vi "ALTS-2015 Show Remaining Time .vi"(8 "error in (no error)":errorcluster, 11 "Time Delay to Restart (Mins)":dbl=2.0 format="%#_13g") -> (0 "error out":errorcluster)   [LabVIEW 2013]
panel:
  in  "Jump Button":bool
  out "Time to be elapsed (in seconds)":u32
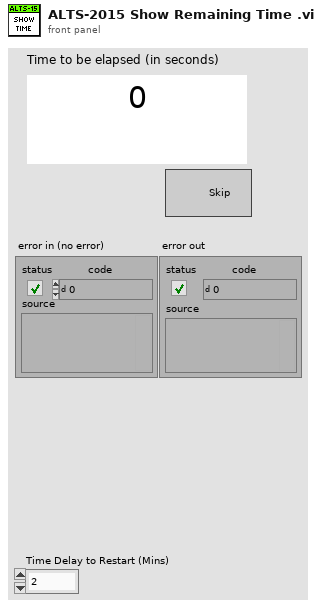
[diagram p1: front panel]
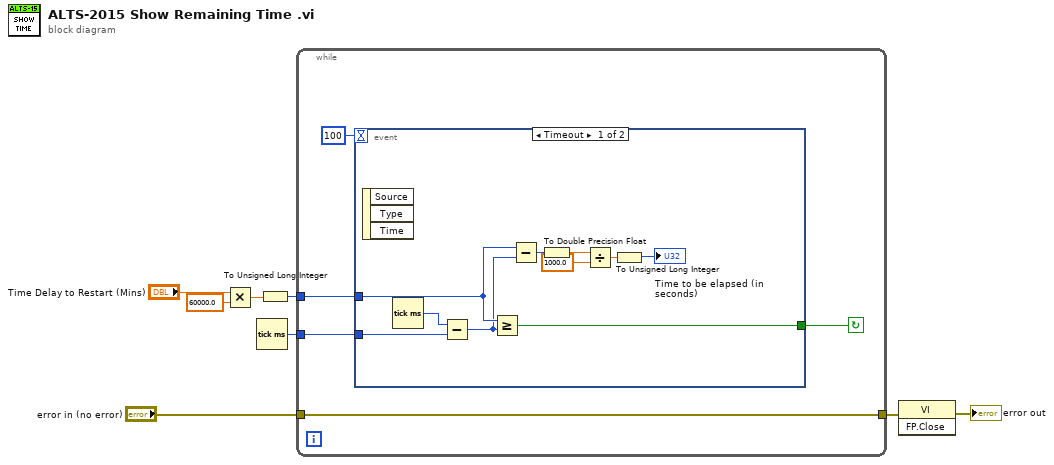
[diagram p0: block diagram]
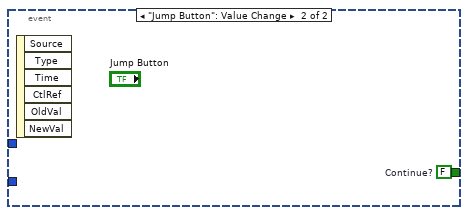
[diagram p2: hidden frame]
diagram:
  n1 = Multiply(x="Time Delay to Restart (Mins)", y=60000.0) -> (x*y=w5:dbl)
  n2 = Tick Count (ms)() -> (millisecond timer value=w8:u32)
  n3 = To Unsigned Long Integer(number=w5) -> (unsigned 32bit integer=w4:u32)
  n4 = while {
    tunnel: w8 -> [w12]
    tunnel: w4 -> [w11]
    tunnel: "error in (no error)" -> [w9]
    tunnel: [w9] -> w3
    stop <- w10 continue-if-true
    n5 = event shown="[0] Timeout" {
      selector: _ -> [_ _]
      dyn-events: _ -> [_ _]
      timeout: 100 -> [_ _]
      tunnel: w12 -> [w22 _]
      tunnel: w11 -> [w20 _]
      tunnel: [w21 w24] -> w10
      event Timeout {
        n6 = event-data() -> ()  [unwired: 1 in, 3 out]
        n7 = Tick Count (ms)() -> (millisecond timer value=w23:u32)
        n8 = Subtract(x=w23, y=w22) -> (x-y=w19:u32)
        n9 = Greater Or Equal?(x=w20, y=w19) -> (x >= y?=w21:bool)
        n10 = Subtract(x=w20, y=w19) -> (x-y=w18:u32)
        n11 = To Double Precision Float(number=w18) -> (double precision float=w15:dbl)
        n12 = Divide(x=w15, y=1000.0) -> (x/y=w16:dbl)
        n13 = To Unsigned Long Integer(number=w16) -> (unsigned 32bit integer=→"Time to be elapsed (in seconds)":u32)
      }
      event "Jump Button": Value Change {
        w24 = FALSE  # Continue?
        n14 = event-data() -> ()  [unwired: 1 in, 6 out]
      }
    }
  }
  n15 = invoke class="VI" method="FP.Close"(error in=w3) -> (error out=→"error out":errorcluster)  [unwired: 2 in, 2 out]
